vi "QueueDequeuWithPayload.vi"(0 "Queue in":refnum<queue>, 1 "error in":errorcluster) -> (2 "Queue out":refnum<queue>, 3 "Action":T1, 4 "Payload":variant, 5 "error out":errorcluster)   [LabVIEW 2017]
uses:
  Action.ctl
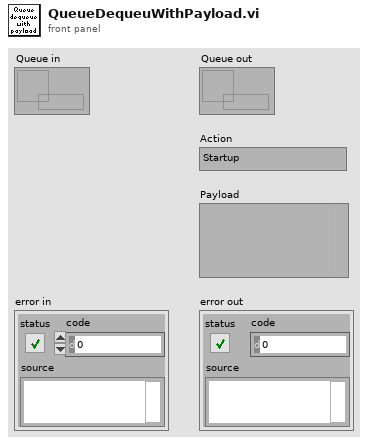
[diagram p1: front panel]
types:
  T1 = typedef "Action.ctl" = enum16{"Startup", "Shutdown", "SaveSettings", "LoadSettings", "InitVNA", "CloseVNA", "InitScan", "IncrementScan", "StopScan", "Target=VNA", "Target=Refrigerator", "Acquire", "Graph", "PNA", "ENA", "ADR", "PPMS"}
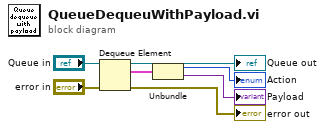
[diagram p0: block diagram]
diagram:
  n1 = Dequeue Element(queue="Queue in", error in (no error)="error in") -> (queue out=→"Queue out":refnum<queue>, element=w1:cluster{"Action":T1, "Payload":variant}, error out=→"error out":errorcluster)  [unwired: 1 in, 1 out]
  n2 = Unbundle(w1) -> ("Action"=→"Action":T1, "Payload"=→"Payload":variant)
